vi "request file path.vi"(8 "error in (no error)":errorcluster, 11 "Data Log in":refnum<class "Data Log.lvclass">) -> (0 "error out":errorcluster, 2 "csv File Path":path caption="selected path", 3 "Data Log out":refnum<class "Data Log.lvclass">)   [LabVIEW 2025, in "Data Log.lvclass"]
uses:
  Data Log.lvclass
  Data Log.lvclass/Data Log.ctl
  <vilib>/Utility/sysdir.llb/System Directory Type.ctl
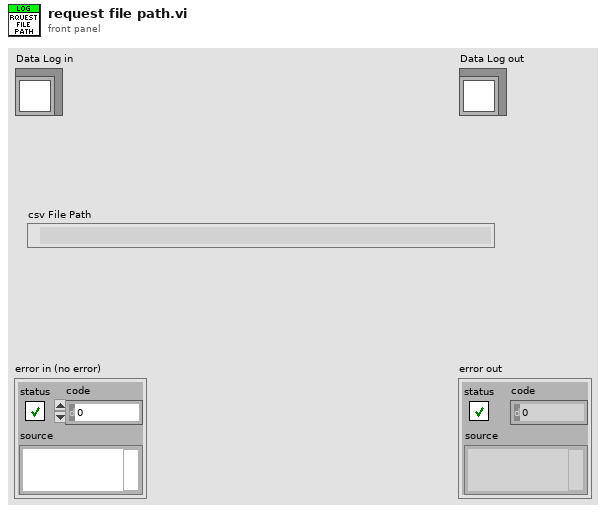
[diagram p1: front panel]
types:
  T1 = typedef "System Directory Type.ctl" = i32
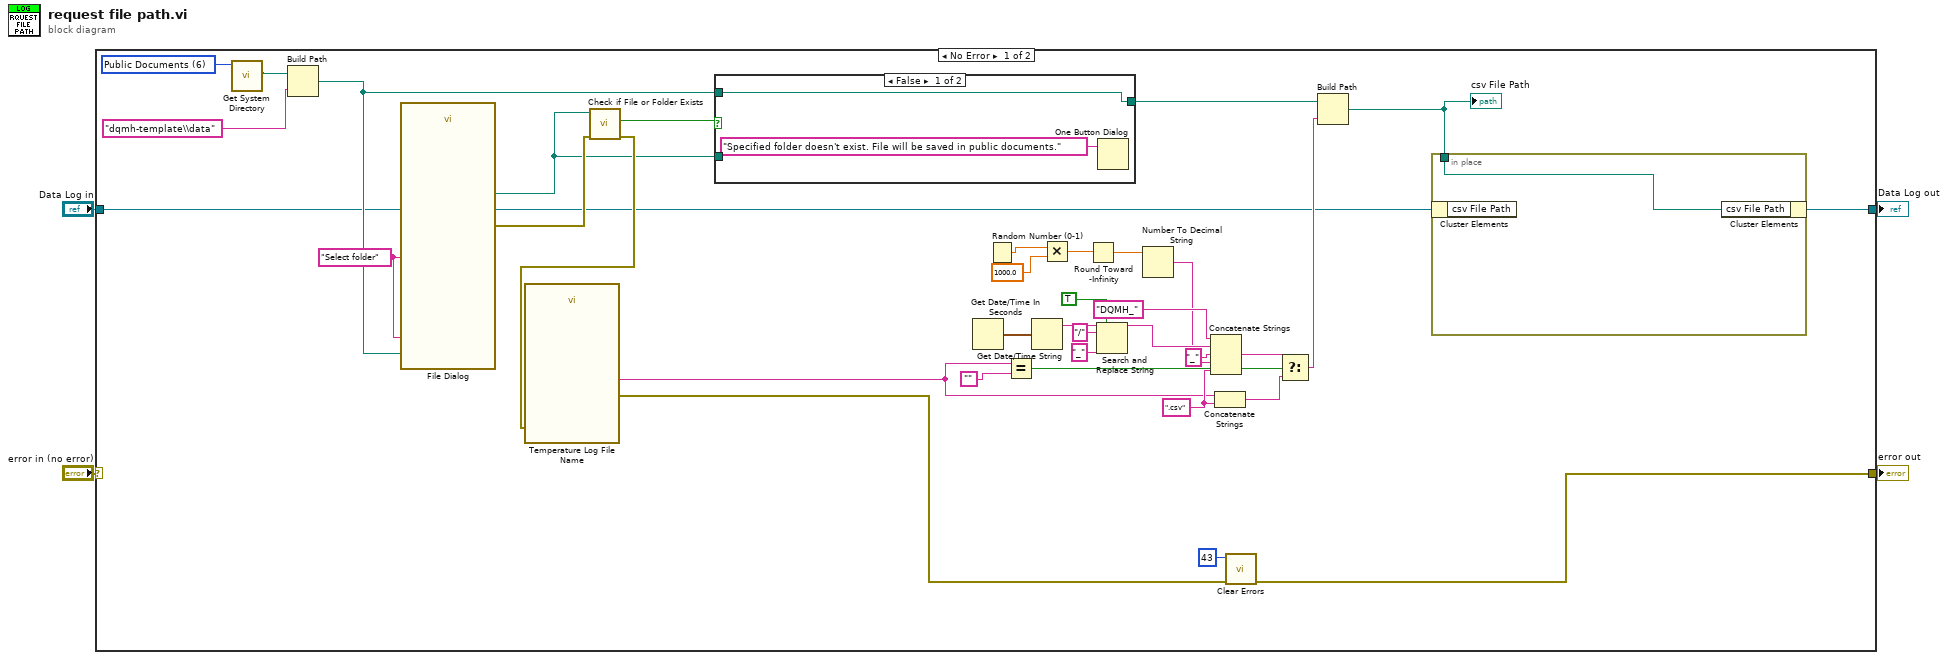
[diagram p0: block diagram]
diagram:
  n1 = case shown="No Error" "error in (no error)" {
    selector: "error in (no error)" -> [_ w46]
    tunnel: [w5 w46] -> w3
    tunnel: [w7 w45] -> w1
    tunnel: "Data Log in" -> [w8 w45]
    frame No Error {
      w19 = ".csv" ("string")
      w14 = "Select folder" ("button label")
      w9 = T1 6 items=["User Home"=0, "User Desktop"=1, "User Documents"=2, "User Application Data"=3, "User Preferences"=4, "User Temporary"=5, "Public Documents"=6, "Public Application Data"=7, "Public Preferences"=8, "Public Cache"=13, "System Core Libraries"=9, "System Installed Libraries"=10, "Application Files"=11, "Boot Volume Root"=12] ("system directory type")
      n2 = call <vilib>:"Get System Directory.vi"("system directory type"=w9) -> ("system directory"=w40:path)  [unwired: 10 in]
      n3 = Build Path(base path=w40, name or relative path="dqmh-template\\data") -> (appended path=w10:path)
      n4 = call "File Dialog"("start path"=w10, "prompt"=w14, "button label"=w14) -> ("selected path"=w11:path, "error out"=w22:errorcluster)  [unwired: 9 in, 2 out]
      n5 = call <vilib>:"Check if File or Folder Exists.vi"("error in (no error)"=w22, "path"=w11) -> ("error out"=w21:errorcluster, "file or folder exists?"=w13:bool)  [unwired: 7 in, 1 out]
      n6 = call "Temperature Log File Name"("error in (no error)"=w21) -> ("File name"=w18:string, "error out"=w15:errorcluster)  [unwired: 16 in, 1 out]
      n7 = case shown="False" w13 {
        tunnel: [w43 w44] -> w12
        tunnel: w11 -> [_ w44]
        tunnel: w10 -> [w43 _]
        frame False {
          n8 = One Button Dialog(message="Specified folder doesn't exist. File will be saved in public documents.") -> ()  [unwired: 1 in, 1 out]
        }
        frame True {
        }
      }
      n9 = Get Date/Time In Seconds() -> (seconds since 1Jan1904=w36:timestamp)
      n10 = Random Number (0-1)() -> (number: 0 to 1=w28:dbl)
      n11 = Equal?(x=w18, y="") -> (x = y?=w37:bool)
      n12 = Get Date/Time String(seconds (now)=w36) -> (date string=w35:string)  [unwired: 2 in, 1 out]
      n13 = Multiply(x=w28, y=1000.0) -> (x*y=w26:dbl)
      n14 = Round Toward -Infinity(1:w26) -> (0:w25:dbl)
      n15 = Search and Replace String(replace all?=TRUE ("replace all? (F)"), input string=w35, search string="/", replace string="_" ("replace string (\"\")")) -> (result string=w32:string)  [unwired: 4 in, 3 out]
      n16 = Number To Decimal String(number=w25) -> (decimal integer string=w24:string)  [unwired: 1 in]
      n17 = Concatenate Strings("DQMH_" ("string"), w32, "_" ("string"), w24, w19) -> (w30:string)
      n18 = Concatenate Strings(w18, w19) -> (w17:string)
      n19 = call <vilib>:"Clear Errors.vi"("error in (no error)"=w15, "specific error code to clear (0: all)"=43) -> ("error out"=w5:errorcluster)  [unwired: 4 in, 1 out]
      n20 = Select(t=w30, s=w37, f=w17) -> (s? t:f=w20:string)
      n21 = Build Path(base path=w12, name or relative path=w20) -> (appended path=w6:path)
      "csv File Path" <- w6
      n22 = in-place {
        in-place-border: w6 -> [w41]
        n23 = in-place-cluster #1(w8) -> ()  [unwired: 1 out]
        n24 = in-place-cluster #1("csv File Path"=w41) -> (w7:refnum<class "Data Log.lvclass">)
      }
    }
    frame Error {
    }
  }
  "error out" <- w3
  "Data Log out" <- w1
